vi "variableExample.vi"() -> ()   [LabVIEW 2014]
panel:
  out "Number of ticks gauge\nIndicator":i32(knob) scale=0.0..100.0
  out "Current Number of Ticks\nIndicator":i32
  out "Tick count array\nIndicator":i32[](array[numeric])
  in  "Initial clock sound\nControl":string="Ting!"
  out "Clock Ticker \nIndicator":string
  in  "Stop Button \nControl":bool
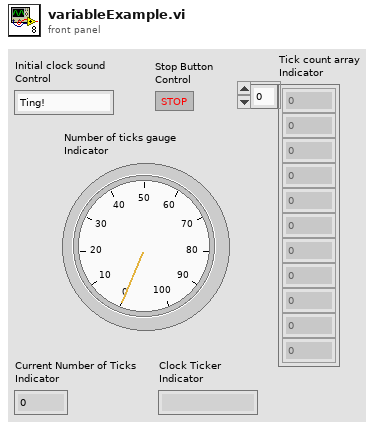
[diagram p1: front panel]
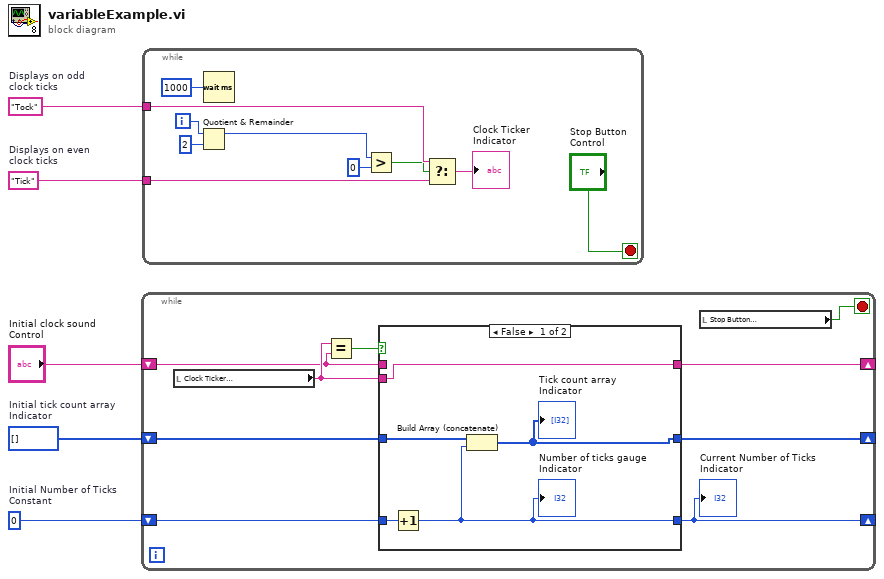
[diagram p0: block diagram]
diagram:
  w1 = i32[] []  # Initial tick count array Indicator
  w2 = 0  # Initial Number of Ticks Constant
  w5 = "Tick"  # Displays on even clock ticks
  w4 = "Tock"  # Displays on odd  clock ticks
  n1 = while {
    shift-right: [w11] -> _
    shift-left: "Initial clock sound\nControl" -> [w8]
    shift-right: [w7] -> _
    shift-left: w2 -> [w12]
    shift-right: [w6] -> _
    shift-left: w1 -> [w10]
    stop <- w13 stop-if-true
    n2 = local read "Clock Ticker \nIndicator"() -> (w9:string)
    n3 = Equal?(x=w9, y=w8) -> (x = y?=w14:bool)
    n4 = case shown="False" w14 {
      tunnel: w12 -> [w19 w22]
      tunnel: [w15 w22] -> w7
      tunnel: w8 -> [_ w21]
      tunnel: [w18 w21] -> w11
      tunnel: w9 -> [w18 _]
      tunnel: w10 -> [w17 w20]
      tunnel: [w16 w20] -> w6
      frame False {
        # "Clock sound strings\ndo not match"
        n5 = Increment(x=w19) -> (x+1=w15:i32)
        "Number of ticks gauge\nIndicator" <- w15
        n6 = Build Array (concatenate) "Build Array"(w17, w15) -> (w16:i32[])
        "Tick count array\nIndicator" <- w16
      }
      frame True {
        # "Clock sound strings\nmatch"
      }
    }
    "Current Number of Ticks\nIndicator" <- w7
    n7 = local read "Stop Button \nControl"() -> (w13:bool)
  }
  n8 = while {
    tunnel: w5 -> [w32]
    tunnel: w4 -> [w31]
    i -> [w30]
    stop <- "Stop Button \nControl" stop-if-true
    n9 = Quotient & Remainder(x=w30, y=2) -> (x-y*floor(x/y)=w28:i32)  [unwired: 1 out]
    n10 = Wait (ms)(milliseconds to wait=u32 1000) -> ()  [unwired: 1 out]
    n11 = Greater?(x=w28, y=0) -> (0:w26:bool)
    n12 = Select(t=w31, s=w26, f=w32) -> (s? t:f=→"Clock Ticker \nIndicator":string)
  }
